vi "ReadState.vi"(8 "error in (no error)":errorcluster, 11 "AdsNET in":refnum<class "AdsNET.lvclass">) -> (0 "error out":errorcluster, 1 "DeviceState":i16, 2 "AdsState":i16(ring) items=["Invalid", "Idle", "Reset", "Init", "Start", "Run", "Stop", "SaveConfig", "LoadConfig", "PowerFailure", "PowerGood", "Error", "Shutdown", "Suspend", "Resume", "Config", "Reconfig", "Maxstates"], 3 "AdsNET out":refnum<class "AdsNET.lvclass">)   [LabVIEW 2016, in "TCatAdsNet.lvlib" / "AdsNET.lvclass"]
uses:
  AdsNET.lvclass
  AdsNET.lvclass/AdsNET.ctl
  C:/Users/Maurizio/Projects/twincat-lv-ads-library/TCatAdsNet Library/TwinCAT.Ads.dll
  TwinCAT.Ads.dll
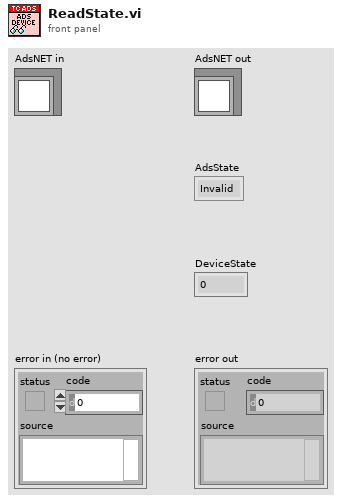
[diagram p1: front panel]
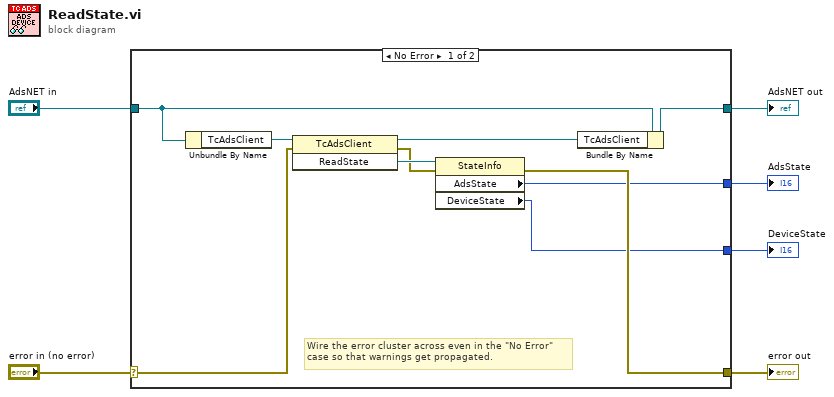
[diagram p0: block diagram]
diagram:
  n1 = case shown="No Error" "error in (no error)" {
    selector: "error in (no error)" -> [w14 w18]
    tunnel: [w9 w18] -> w5
    tunnel: [w13 w17] -> w3
    tunnel: "AdsNET in" -> [w16 w17]
    tunnel: [w8 _] -> w2
    tunnel: [w7 _] -> w1
    frame No Error {
      # "Wire the error cluster across even in the \"No Error\"\ncase so that warnings get propagated."
      n2 = Unbundle By Name(w16) -> ("TcAdsClient"=w15:refnum<k24>)
      n3 = invoke class="TcAdsClient" method="ReadState"(reference=w15, error in=w14) -> (reference out=w12:refnum<k24>, error out=w10:errorcluster, "ReadState"=w11:refnum<k24>)  [unwired: 1 in]
      n4 = property class="StateInfo"(reference=w11, error in=w10) -> (error out=w9:errorcluster, "AdsState"=w8:i16, "DeviceState"=w7:i16)  [unwired: 1 out]
      n5 = Bundle By Name(cluster=w16, "TcAdsClient"=w12) -> (w13:refnum<class "AdsNET.lvclass">)
    }
    frame Error {
    }
  }
  "error out" <- w5
  "AdsNET out" <- w3
  "DeviceState" <- w1
  "AdsState" <- w2
